vi "NormaliseProfile.vi"(5 "ResampleHeights":dbl[](array[numeric])=[25.4, 38.1, 50.8, 76.2, 101.6, 127.0, 152.4, 203.2, 254.0, 304.8, 406.4, 508.0, 609.6, 812.8, 1219.2, 1524.0], 6 "Zref":dbl=508.0 min=0.0, 7 "ResampleToN":i32, 10 "UzClusterIn":cluster{dbl[], dbl[]}, 11 "Resampler":T1) -> (1 "U(Zref)":dbl, 3 "UzClusterOutput":cluster{dbl[], dbl[]})   [LabVIEW 2014]
uses:
  Resampler.ctl
  <vilib>/Analysis/NI_AALPro.lvlib
  <vilib>/gmath/NI_Gmath.lvlib
panel:
  in  "Interpolation":i32(ring)=1 items=["nearest", "linear", "spline", "cubic Hermite", "Lagrange"]
  out "UzClusterNormalisedResampled":cluster{dbl[], dbl[]}
  out "UzClusterNormalised":cluster{dbl[], dbl[]}
  in  "binTolerance":dbl=10.0
  out "firstBelow":dbl
  out "firstAbove":dbl
  out "XY Graph":cluster{dbl[], dbl[]}[](graph)
  # "Fit using values at  measurement Z heights"
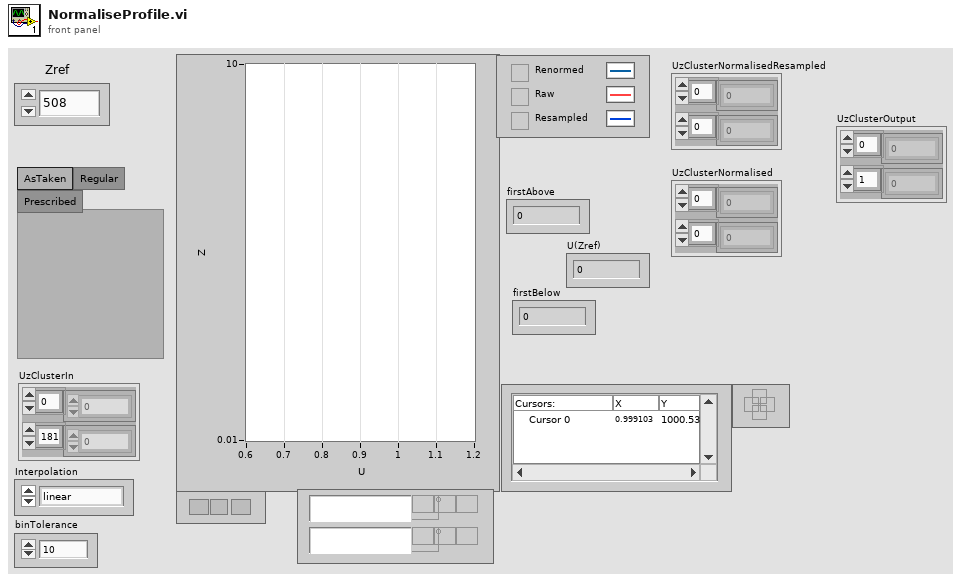
[diagram p1: front panel]
types:
  T1 = typedef "Resampler.ctl" = enum32{"AsTaken", "Regular", "Prescribed"}
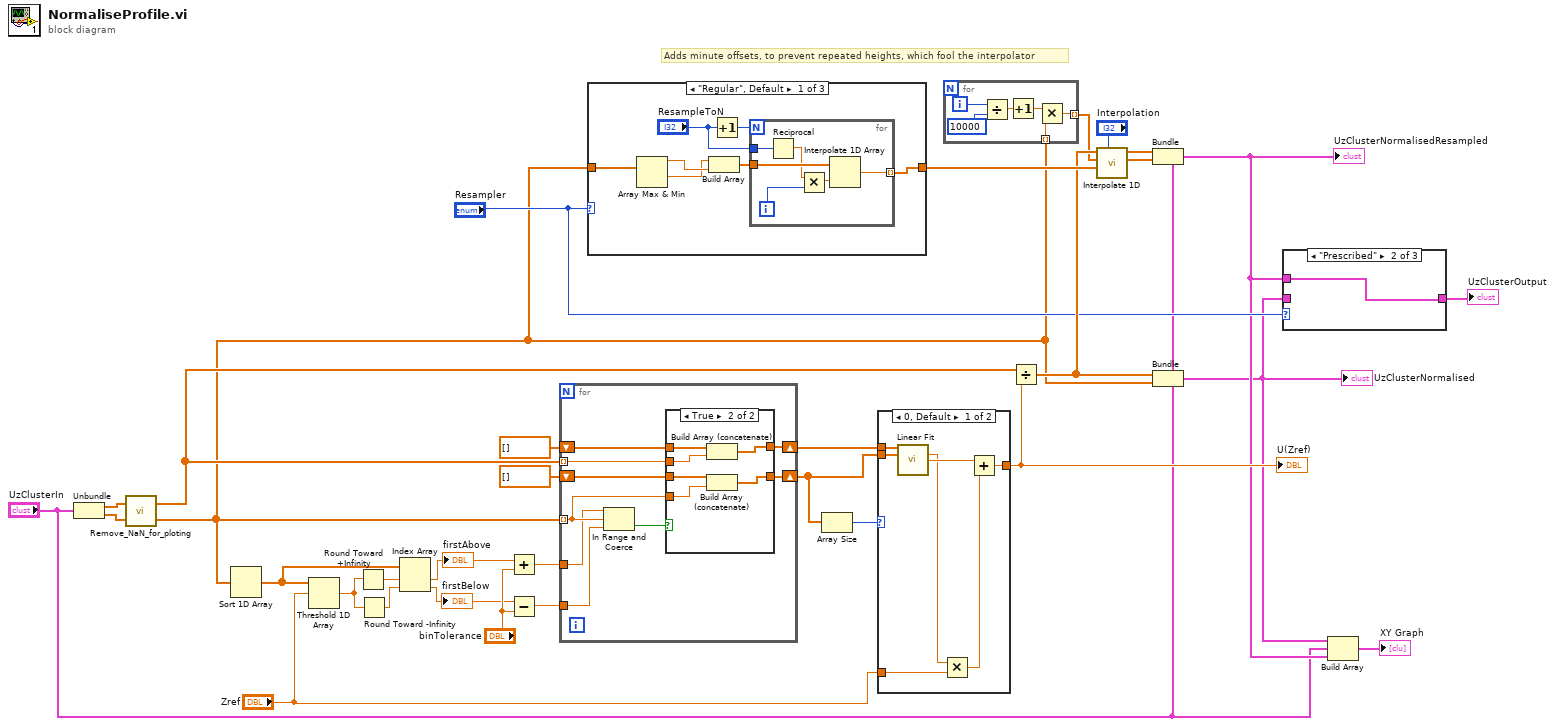
[diagram p0: block diagram]
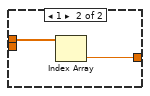
[diagram p4: hidden frame]
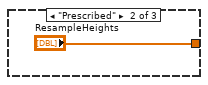
[diagram p5: hidden frame]
diagram:
  # "Adds minute offsets, to prevent repeated heights, which fool the interpolator"
  n1 = Unbundle("UzClusterIn") -> (w19:dbl[], w20:dbl[])
  n2 = call "Remove_NaN_for_ploting.vi"("Array 2"=w20, "Array 1"=w19) -> ("Array 2 Out"=w6:dbl[], "Array 1 Out"=w18:dbl[])
  n3 = Sort 1D Array(array=w6) -> (sorted array=w31:dbl[])
  n4 = Threshold 1D Array(2:"Zref", 3:w31) -> (0:w32:dbl)  [unwired: 1 in]
  n5 = Round Toward +Infinity(x=w32) -> (ceil(x): smallest int >= x=w30:dbl)
  n6 = Round Toward -Infinity(1:w32) -> (0:w29:dbl)
  n7 = Index Array(array=w31, index #1=w30, index #2=w29) -> (element #1=w13:dbl, element #2=w12:dbl)
  "firstAbove" <- w13
  "firstBelow" <- w12
  n8 = Add(x=w13, y="binTolerance") -> (x+y=w27:dbl)
  n9 = Subtract(x=w12, y="binTolerance") -> (x-y=w26:dbl)
  n10 = for {
    tunnel: w18 -> [w40] mode=indexing
    tunnel: w6 -> [w41] mode=indexing
    tunnel: w27 -> [w35]
    tunnel: w26 -> [w34]
    shift-right: [w39] -> w25
    shift-left: dbl[] [] -> [w38]
    shift-right: [w36] -> w8
    shift-left: dbl[] [] -> [w37]
    n11 = In Range and Coerce(upper limit=w35, x=w41, lower limit=w34) -> (In Range?=w33:bool)  [unwired: 1 out]
    n12 = case shown="True" w33 {
      tunnel: w41 -> [_ w49]
      tunnel: w40 -> [_ w48]
      tunnel: [w43 w47] -> w39
      tunnel: w38 -> [w43 w46]
      tunnel: w37 -> [w42 w45]
      tunnel: [w42 w44] -> w36
      frame False {
      }
      frame True {
        n13 = Build Array (concatenate)(w46, w48) -> (w47:dbl[])
        n14 = Build Array (concatenate)(w45, w49) -> (w44:dbl[])
      }
    }
  }
  n15 = case shown="\"Regular\", Default" "Resampler" {
    tunnel: [w52 "ResampleHeights" w64] -> w15
    tunnel: w6 -> [w50 _ w64]
    frame "Regular", Default {
      n16 = Array Max & Min(array=w50) -> (max value=w54:dbl, min value=w53:dbl)  [unwired: 2 out]
      n17 = Build Array(w53, w54) -> (w56:dbl[])
      n18 = Increment(x="ResampleToN") -> (x+1=w51:i32)
      n19 = for {
        N: w51 -> [_]
        tunnel: w56 -> [w62]
        tunnel: "ResampleToN" -> [w61]
        tunnel: [w58] -> w52 mode=indexing
        i -> [w57]
        n20 = Reciprocal(x=w61) -> (1/x=w59:dbl)
        n21 = Multiply(x=w59, y=w57) -> (x*y=w60:dbl)
        n22 = Interpolate 1D Array(1:w60, 2:w62) -> (0:w58:dbl)
      }
    }
    frame "Prescribed" {
    }
    frame "AsTaken" {
    }
  }
  n23 = Array Size(array=w8) -> (size(s)=w11:i32)
  n24 = case shown="0, Default" w11 {
    tunnel: w25 -> [w71 w73]
    tunnel: "Zref" -> [w68 _]
    tunnel: [w66 w72] -> w24
    tunnel: w8 -> [w65 _]
    frame 0, Default {
      n25 = call <vilib>:"Linear Fit.vi"("Y"=w71, "X"=w65) -> ("slope"=w69:dbl, "intercept"=w70:dbl)  [unwired: 9 in, 3 out]
      n26 = Multiply(x=w69, y=w68) -> (x*y=w67:dbl)
      n27 = Add(x=w70, y=w67) -> (x+y=w66:dbl)
    }
    frame 1 {
      n28 = Index Array(array=w73) -> (element=w72:dbl)  [unwired: 1 in]
    }
  }
  "U(Zref)" <- w24
  n29 = for {
    tunnel: [w74] -> w7 mode=indexing
    tunnel: w6 -> [w75] mode=indexing
    i -> [w79]
    n30 = Divide(x=w79, y=10000) -> (x/y=w77:dbl)
    n31 = Increment(x=w77) -> (x+1=w76:dbl)
    n32 = Multiply(x=w76, y=w75) -> (x*y=w74:dbl)
  }
  n33 = Divide(x=w18, y=w24) -> (x/y=w14:dbl[])
  n34 = call <vilib>:"Interpolate 1D.vi"("method"="Interpolation", "xi"=w15, "X"=w7, "Y"=w14) -> ("xi used"=w5:dbl[], "yi"=w16:dbl[])  [unwired: 5 in, 1 out]
  n35 = Bundle(cluster="UzClusterIn", w16, w5) -> (w3:cluster{dbl[], dbl[]})
  "UzClusterNormalisedResampled" <- w3
  n36 = Bundle(cluster="UzClusterIn", w14, w6) -> (w1:cluster{dbl[], dbl[]})
  "UzClusterNormalised" <- w1
  n37 = case shown="\"Prescribed\"" "Resampler" {
    tunnel: [w80 w81 w82] -> w9
    tunnel: w3 -> [w80 w81 _]
    tunnel: w1 -> [_ _ w82]
    frame "Regular", Default {
    }
    frame "Prescribed" {
    }
    frame "AsTaken" {
    }
  }
  "UzClusterOutput" <- w9
  n38 = Build Array(w1, "UzClusterIn", w3) -> (→"XY Graph":cluster{dbl[], dbl[]}[])
